vi "Get Message Field Info.vi"(8 "error in (no error)":errorcluster, 11 "Message Field ref in":u64) -> (0 "error out":errorcluster, 2 "Field Info":T1={"Field Name"="", "Embedded Message Name"="", "Protobuf Index"=1, "MessageElementType"=enum."StringValue", "Repeated"=FALSE}, 3 "Message Field ref out":u64)   [LabVIEW 2019, in "gRPC Scripting Tools.lvlib"]
uses:
  gRPC Scripting Tools.lvlib
  TypeDefs/Message Element Metadata (Scripting).ctl
  TypeDefs/Message Element Type.ctl
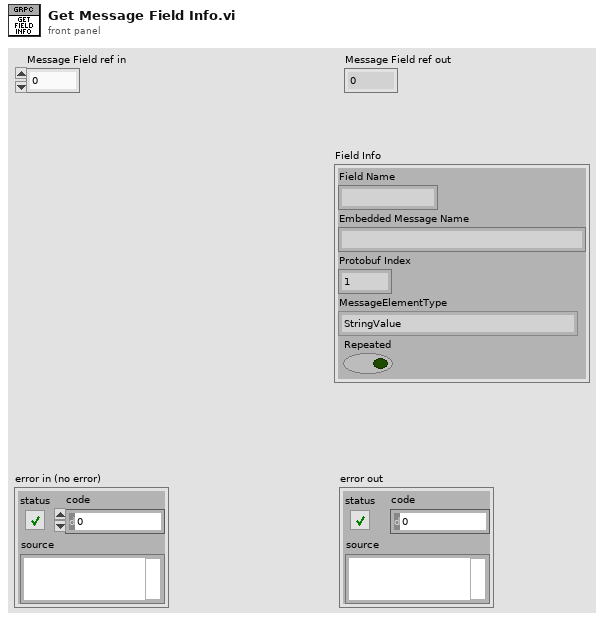
[diagram p1: front panel]
types:
  T1 = typedef "gRPC Scripting Tools.lvlib/Message Element Metadata (Scripting).ctl" = cluster{"Field Name":string, "Embedded Message Name":string, "Protobuf Index":i32, "MessageElementType":T2, "Repeated":bool}
  T2 = typedef "gRPC Scripting Tools.lvlib/Message Element Type.ctl" = enum32{"Int32Value", "FloatValue", "DoubleValue", "BoolValue", "StringValue", "MessageValue", "Int64Value", "UInt32Value", "UInt64Value", "EnumValue", "Bytes", "Fixed64", "Fixed32", "SFixed64", "SFixed32", "SInt64", "SInt32"}
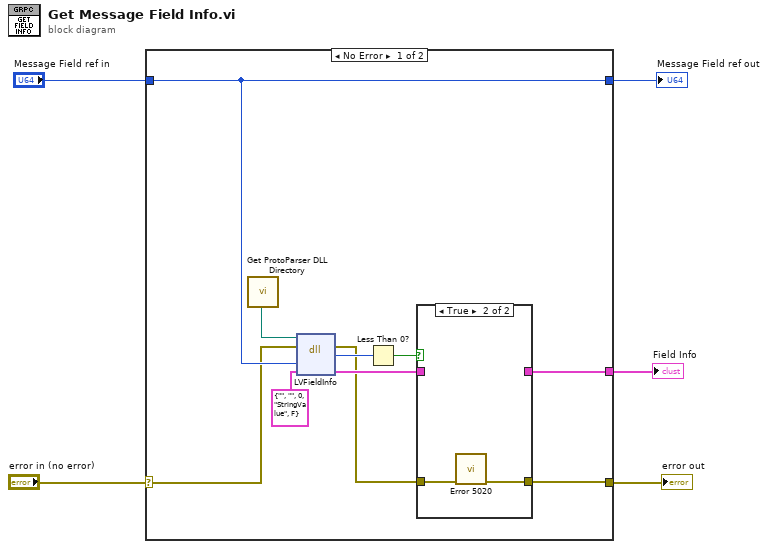
[diagram p0: block diagram]
diagram:
  n1 = case shown="No Error" "error in (no error)" {
    selector: "error in (no error)" -> [w14 w21]
    tunnel: "Message Field ref in" -> [w15 w20]
    tunnel: [w15 w20] -> w3
    tunnel: [w6 w21] -> w2
    tunnel: [w10 _] -> w1
    frame No Error {
      n2 = call "Get ProtoParser DLL Directory.vi"() -> ("Proto Parser Directory"=w12:path)
      n3 = dll-call lib="C:/Users/XEnderMD/Desktop/LV gRPC/labview source/gRPC Scripting Tools/Proto Parser API/dll/labview_grpc_generator.dll" fn="LVFieldInfo"(path in=w12, error in=w14, "field"=w15, "fieldInfo"=T1 {"Field Name"="", "Embedded Message Name"="", "Protobuf Index"=0, "MessageElementType"=enum."StringValue", "Repeated"=FALSE} ("MessageElementMetadata")) -> (error out=w7:errorcluster, "return type"=w9:i32, "fieldInfo"=w11:T1)  [unwired: 2 in, 1 out]
      n4 = Less Than 0?(x=w9) -> (x < 0?=w8:bool)
      n5 = case shown="True" w8 {
        tunnel: w11 -> [w16 _]
        tunnel: [w16 _] -> w10
        tunnel: w7 -> [w17 w19]
        tunnel: [w17 w18] -> w6
        frame False {
        }
        frame True {
          n6 = call "Error 5020.vi"("error in (no error)"=w19) -> ("error out"=w18:errorcluster)  [unwired: 10 in]
        }
      }
    }
    frame Error {
    }
  }
  "Message Field ref out" <- w3
  "error out" <- w2
  "Field Info" <- w1
